vi "Actor Core.vi"(8 "error in":errorcluster, 11 "Camera Tester in":refnum<class "Camera Tester.lvclass">) -> (0 "error out":errorcluster, 3 "Actor out":refnum<class "Actor.lvclass">)   [LabVIEW 2014, in "Camera Tester.lvlib" / "Camera Tester.lvclass"]
doc: "(<B>Filename</B>: Actor Framework.lvlib:Actor.lvclass:Actor Core.vi)\n\nReceives messages to the actor, reacts to them, and initiates any error handling that may shut the actor down.\n\nDescendant classes may override this VI to append parallel tasks for the actor to complete while it handles messages. Overrides use the Call Parent Method node."
uses:
  Camera Tester.lvclass
  <vilib>/ActorFramework/Actor/Actor.lvclass
  <vilib>/userdefined/High Color/IMAQdx.ctl
  <vilib>/ActorFramework/Actor/Actor.lvclass/Actor.ctl
  <vilib>/ActorFramework/Message Enqueuer/Message Enqueuer.lvclass/Message Enqueuer.ctl
  Viewable Actor/ViewableActor/ViewableActor.lvclass/ViewableActor.ctl
  Camera Tester.lvclass/Camera Tester.ctl
  Camera Tester Messages/Start Camera Msg/Start Camera Msg.lvclass/Start Camera Msg.ctl
  Viewable Actor/ViewableActor/Read Stop Event.vi
  <vilib>/ActorFramework/Message Enqueuer/Init from Existing Queue.vi
  <vilib>/ActorFramework/Message Enqueuer/Enqueue.vi
  <vilib>/ActorFramework/Message Priority Queue/Priority Enqueue.vi
  <vilib>/ActorFramework/Message Enqueuer/Message Enqueuer.lvclass
  <vilib>/ActorFramework/Stop Msg/Stop Msg.lvclass
  Camera Tester Messages/Start Camera Msg/Start Camera Msg.lvclass
  Camera Tester Messages/open camera settings Msg/open camera settings Msg.lvclass
  Viewable Actor/ViewableActor Messages/Open Front Panel Msg/Open Front Panel Msg.lvclass
  Viewable Actor/ViewableActor/ViewableActor.lvclass
panel:
  out "Image display":T1(plugin-control)
  in  "Start Camera":bool
  in  "Settings":bool
  in  "Syslog Config":path=path "Z:/HIJ_Vision_Project/Submodules/HIJ Vision/Camera Actors/Camera Tester/Camera Tester/config.cfg"
  in  "IMAQdx Session":T2="cam0"
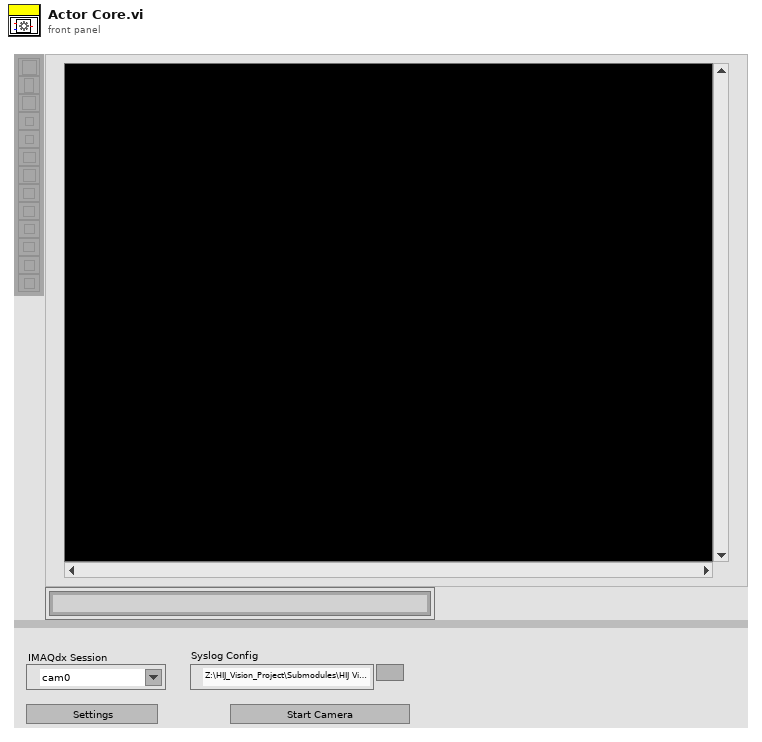
[diagram p1: front panel]
types:
  T1 = typedef "IMAQ Image.ctl" = refnum<image>
  T2 = typedef "IMAQdx.ctl" = refnum<k21>
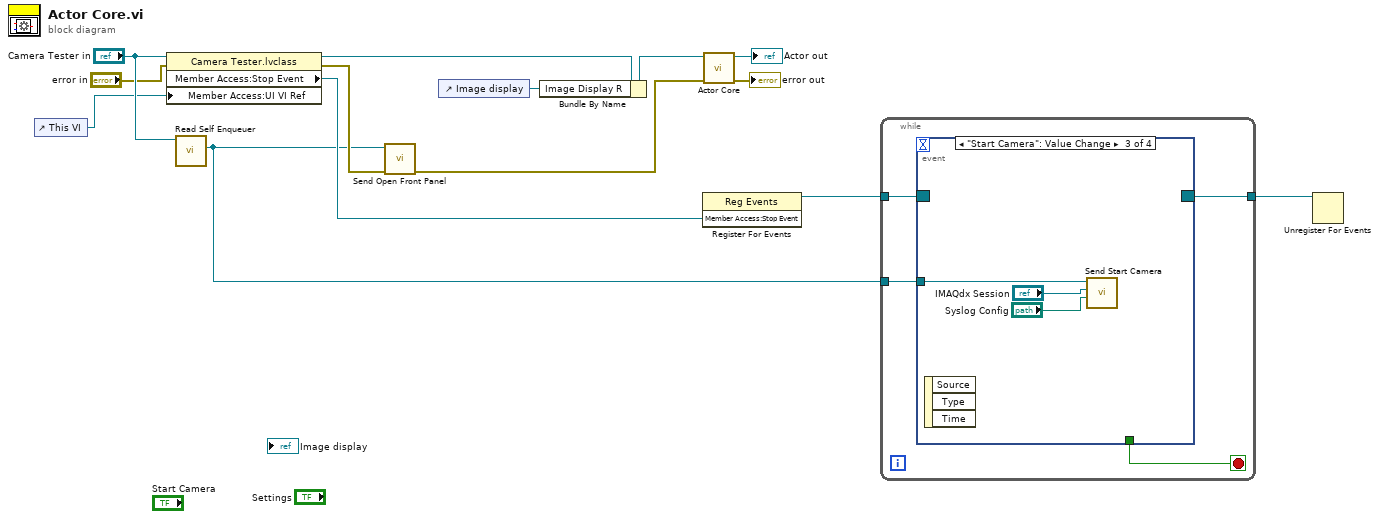
[diagram p0: block diagram]
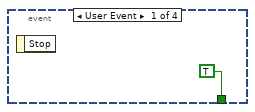
[diagram p2: hidden frame]
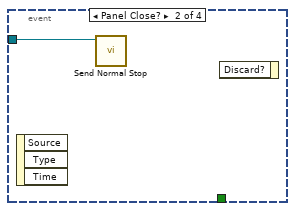
[diagram p3: hidden frame]
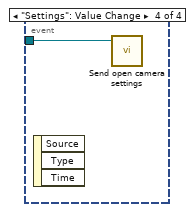
[diagram p4: hidden frame]
diagram:
  n1 = control-ref of="This VI"() -> (w6:refnum<vi>)
  n2 = property class="Camera Tester.lvclass"(reference="Camera Tester in", error in="error in", "Member Access:UI VI Ref"=w6) -> (reference out=w7:refnum<class "Camera Tester.lvclass">, error out=w5:errorcluster, "Member Access:Stop Event"=w11:refnum<user-event>)
  n3 = call <vilib>:"Read Self Enqueuer.vi"("Actor"="Camera Tester in") -> ("Self Enqueuer"=w3:refnum<class "Message Enqueuer.lvclass">)  [unwired: 10 in]
  n4 = call "Send Open Front Panel.vi"("error in (no error)"=w5, "Message Enqueuer"=w3) -> ("error out"=w4:errorcluster)  [unwired: 8 in, 1 out]
  n5 = control-ref of="Image display"() -> (w1:refnum<vi>)
  n6 = Bundle By Name(cluster=w7, "Image Display R"=w1) -> (w2:refnum<class "Camera Tester.lvclass">)
  n7 = register-events(w11) -> (reference out=w10:refnum<event-registration>)  [unwired: 2 in, 1 out]
  n8 = call-parent "Actor Core.vi"("error in"=w4, "Actor in"=w2) -> ("error out"=→"error out":errorcluster, "Actor out"=→"Actor out":refnum<class "Actor.lvclass">)  [unwired: 8 in]
  n9 = while {
    tunnel: w10 -> [w18]
    tunnel: w3 -> [w16]
    tunnel: [w15] -> w9
    stop <- w17 stop-if-true
    n10 = event shown="[2] \"Start Camera\": Value Change" {
      selector: w18 -> [_ _ _ _]
      dyn-events: [_ _ _ _] -> w15
      timeout: _ -> [_ _ _ _]
      tunnel: [TRUE _ _ _] -> w17
      tunnel: w16 -> [_ w20 w23 w24]
      event User Event {
        n11 = event-data() -> ()  [unwired: 1 in, 1 out]
      }
      event Panel Close? {
        n12 = event-data() -> ()  [unwired: 1 in, 3 out]
        n13 = call <vilib>:"Send Normal Stop.vi"("Message Enqueuer"=w20) -> ()  [unwired: 10 in, 1 out]
        n14 = event-data() -> ()  [unwired: 2 in, 1 out]
      }
      event "Start Camera": Value Change {
        n15 = event-data() -> ()  [unwired: 1 in, 3 out]
        n16 = call "Send Start Camera.vi"("Config file"="Syslog Config", "IMAQdx Session"="IMAQdx Session", "Message Enqueuer"=w23) -> ()  [unwired: 7 in, 2 out]
      }
      event "Settings": Value Change {
        n17 = event-data() -> ()  [unwired: 1 in, 3 out]
        n18 = call "Send open camera settings.vi"("Message Enqueuer"=w24) -> ()  [unwired: 9 in, 2 out]
      }
    }
  }
  n19 = Unregister For Events(event registration refnum=w9) -> ()  [unwired: 1 in, 1 out]
